vi "Read IPS PSU Group Current Voltage.vi"(6 "Axis":T1, 8 "error in (no error)":errorcluster, 11 "Instrument.OxfordVRM in":refnum<class "Instrument.OxfordVRM.lvclass">) -> (0 "error out":errorcluster, 1 "Voltage (V)":dbl, 2 "Current (A)":dbl, 3 "Instrument.OxfordVRM out":refnum<class "Instrument.OxfordVRM.lvclass">)   [LabVIEW 2016, in "Instrument.OxfordVRM.lvclass"]
uses:
  Instrument.OxfordVRM.lvclass
  <instrlib>/Mercury iXX/Mercury iXX.lvlib
  <instrlib>/Mercury iXX/Public/Libraries/Magnet/Signals/Read/Current (Read).vi
  <instrlib>/Mercury iXX/Public/Libraries/Magnet.lvlib
  <instrlib>/Mercury iXX/Public/Libraries/Magnet/Signals/Read/Voltage (Read).vi
  <instrlib>/Mercury iXX/Public/Libraries/Magnet/Open/Open Magnet Device.vi
  <userlib>/LevyLab/Levylab Instruments/Instrument Types/Cryostat/Typedefs/Magnet Axis--Enum.ctl
  <userlib>/LevyLab/Levylab Instruments/Instrument Types/Cryostat/Instrument.Cryostat.lvclass
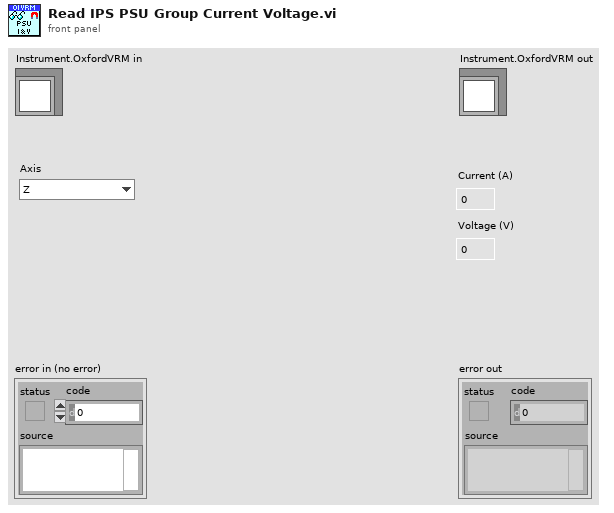
[diagram p1: front panel]
types:
  T1 = typedef "Instrument.Cryostat.lvclass/Magnet Axis--Enum.ctl" = enum16{"Z", "X", "Y"}
  T2 = typedef "Mercury iXX.lvlib/Mercury Reference.ctl" = cluster{"Comms":refnum<visa-resource-name>, "Device ID":string[], "Comms Layer":T3, "Command":string, "Query reference":T4}
  T3 = typedef "Mercury iXX.lvlib/Comms Transport Layer.ctl" = enum16{"Ethernet TCP/IP", "USB", "ISOBus - RS-232", "GPIB"}
  T4 = typedef "Mercury iXX.lvlib/Query Dynamic Reference.ctl" = refnum<vi>
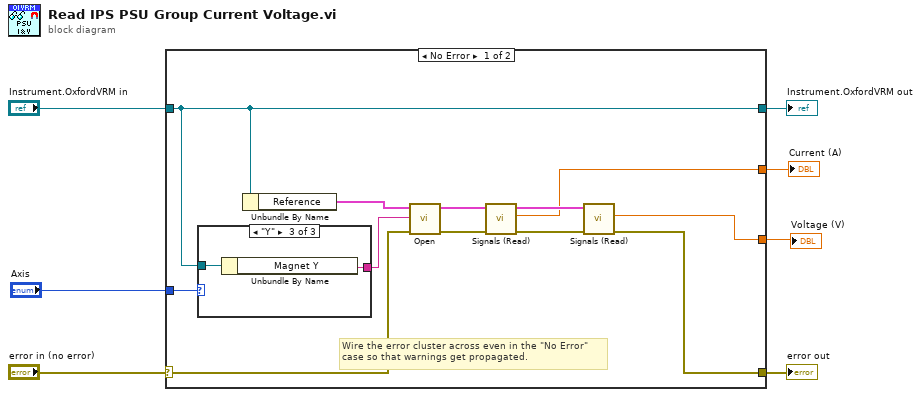
[diagram p0: block diagram]
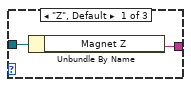
[diagram p2: hidden frame]
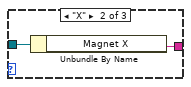
[diagram p3: hidden frame]
diagram:
  n1 = case shown="No Error" "error in (no error)" {
    selector: "error in (no error)" -> [w16 w27]
    tunnel: [w11 w27] -> w6
    tunnel: [w9 w26] -> w4
    tunnel: "Instrument.OxfordVRM in" -> [w9 w26]
    tunnel: [w12 _] -> w3
    tunnel: [w13 _] -> w2
    tunnel: "Axis" -> [w10 _]
    frame No Error {
      # "Wire the error cluster across even in the \"No Error\"\ncase so that warnings get propagated."
      n2 = case shown="\"Y\"" w10 {
        tunnel: [w21 w23 w24] -> w8
        tunnel: w9 -> [w20 w22 w25]
        frame "Z", Default {
          n3 = Unbundle By Name(w20) -> ("Magnet Z"=w21:string)
        }
        frame "X" {
          n4 = Unbundle By Name(w22) -> ("Magnet X"=w23:string)
        }
        frame "Y" {
          n5 = Unbundle By Name(w25) -> ("Magnet Y"=w24:string)
        }
      }
      n6 = Unbundle By Name(w9) -> ("Reference"=w17:T2)
      n7 = call-poly <instrlib>:"Open.vi"("error in (no error)"=w16, "Device Identifier"=w8, "Mercury Reference In"=w17) -> ("error out"=w19:errorcluster, "Mercury Reference Out"=w18:T2)  [unwired: 7 out]
      n8 = call-poly <instrlib>:"Signals (Read).vi"("error in"=w19, "Mercury Reference In"=w18) -> ("error out"=w15:errorcluster, "Current"=w12:dbl, "Mercury Reference Out"=w14:T2)  [unwired: 1 in, 6 out]
      n9 = call-poly <instrlib>:"Signals (Read).vi"("error in"=w15, "Mercury Reference In"=w14) -> ("error out"=w11:errorcluster, "Voltage"=w13:dbl)  [unwired: 1 in, 7 out]
    }
    frame Error {
    }
  }
  "error out" <- w6
  "Instrument.OxfordVRM out" <- w4
  "Current (A)" <- w3
  "Voltage (V)" <- w2
